vi "Write IP Address.vi"(7 "Unit ID":u8, 8 "error in (no error)":errorcluster, 9 "Port":u16, 10 "IP Address":string, 11 "IgusMotorDrive in":refnum<class "IgusMotorDrive.lvclass">) -> (0 "error out":errorcluster, 3 "IgusMotorDrive out":refnum<class "IgusMotorDrive.lvclass">)   [LabVIEW 2016, in "IgusMotorDrive.lvclass"]
doc: "This VI sets the address details of the drive, including IP address, port and unit ID.\n\n<b>Copyright (C) 2018 Control Software Solutions Limited.\nAll rights reserved. </b>"
uses:
  IgusMotorDrive.lvclass
  IgusMotorDrive.lvclass/IgusMotorDrive.ctl
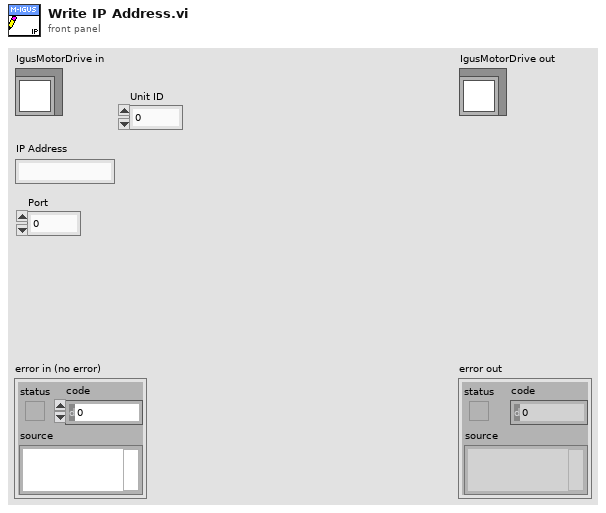
[diagram p1: front panel]
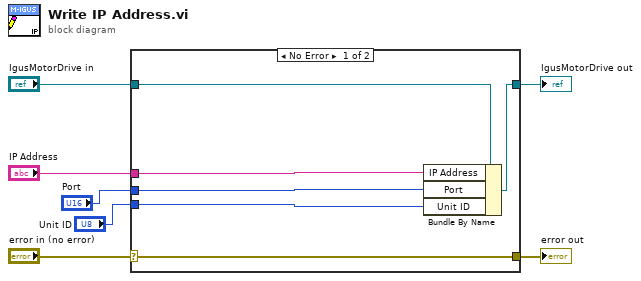
[diagram p0: block diagram]
diagram:
  n1 = case shown="No Error" "error in (no error)" {
    selector: "error in (no error)" -> [w13 w14]
    tunnel: [w13 w14] -> w6
    tunnel: [w11 w15] -> w4
    tunnel: "IgusMotorDrive in" -> [w12 w15]
    tunnel: "IP Address" -> [w10 _]
    tunnel: "Port" -> [w9 _]
    tunnel: "Unit ID" -> [w8 _]
    frame No Error {
      n2 = Bundle By Name(cluster=w12, "IP Address"=w10, "Port"=w9, "Unit ID"=w8) -> (w11:refnum<class "IgusMotorDrive.lvclass">)
    }
    frame Error {
    }
  }
  "error out" <- w6
  "IgusMotorDrive out" <- w4
